vi "Main.vi"   [LabVIEW 2020]
uses:
  Actor/Caller/Caller.lvclass
  C:/Program Files/National Instruments/LabVIEW 2020/vi.lib/ActorFramework/Actor/Actor.lvclass
  <vilib>/ActorFramework/Actor/Actor.lvclass
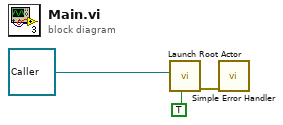
[diagram p0: block diagram]
diagram:
  n1 = call <vilib>:"Launch Root Actor.vi"("Open Actor Core front panel? (F)"=TRUE, "Actor"=refnum<class "Caller.lvclass"> refnum ("Caller.lvlib:Caller.lvclass")) -> ("error out"=w3:errorcluster)  [unwired: 8 in, 1 out]
  n2 = call <vilib>:"Simple Error Handler.vi"("error in (no error)"=w3) -> ()  [unwired: 4 in, 5 out]
